vi "Read Configure.vi"(8 "error in (no error)":errorcluster, 11 "Gluing Procedure in":refnum<class "Gluing Procedure.lvclass">) -> (0 "error out":errorcluster, 2 "Configure":T1={"Has been run?"=FALSE, "Active Paths"=[TRUE, TRUE, TRUE, TRUE], "Glue Pathways"=[{"HDI Slot "=0, "Stamp Slot"=0, "Glue Slot"=0, "Weight Slot"=0, "BBM Slot"=0}, {"HDI Slot "=1, "Stamp Slot"=1, "Glue Slot"=1, "Weight Slot"=1, "BBM Slot"=1}, {"HDI Slot "=2, "Stamp Slot"=2, "Glue Slot"=2, "Weight Slot"=2, "BBM Slot"=2}, {"HDI Slot "=3, "Stamp Slot"=3, "Glue Slot"=3, "Weight Slot"=3, "BBM Slot"=3}], "Chuck Module Used for BBM:"=0} {"Chuck Module Used for BBM:" items=["Chuck 1", "Chuck 2", "Chuck 3", "Chuck 4"]; "Glue Pathways"."BBM Slot" items=["Slot 1", "Slot 2", "Slot 3", "Slot 4"]; "Glue Pathways"."Weight Slot" items=["Slot 1", "Slot 2", "Slot 3", "Slot 4"]; "Glue Pathways"."Glue Slot" items=["Slot 1", "Slot 2", "Slot 3", "Slot 4"]; "Glue Pathways"."Stamp Slot" items=["Slot 1", "Slot 2", "Slot 3", "Slot 4"]; "Glue Pathways"."HDI Slot" items=["Slot 1", "Slot 2", "Slot 3", "Slot 4"]}, 3 "Gluing Procedure out":refnum<class "Gluing Procedure.lvclass">)   [LabVIEW 2011, in "Gluing Procedure.lvclass"]
uses:
  Gluing Procedure.lvclass
  Type Definitions/Configure.ctl
  UI typedefs/Active Paths.ctl
  UI typedefs/Glue Paths.ctl
  UI typedefs/Glue Path.ctl
  UI typedefs/BBM Chuck Used.ctl
  Gluing Procedure.lvclass/Gluing Procedure.ctl
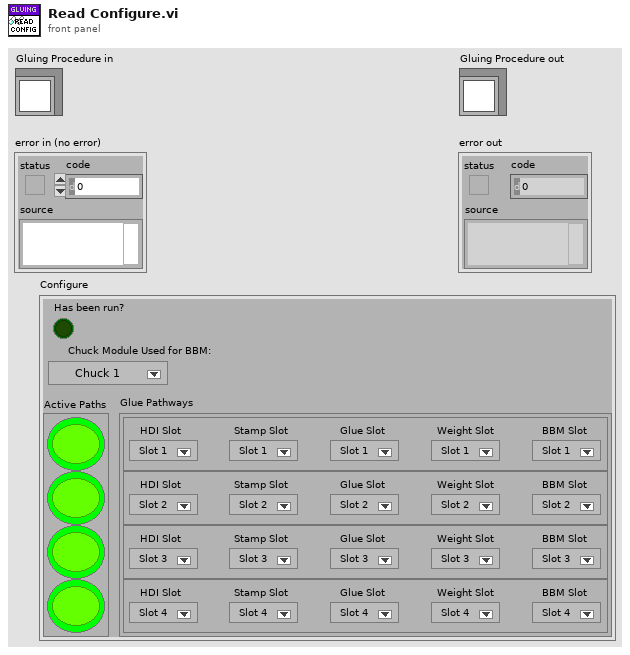
[diagram p1: front panel]
types:
  T1 = typedef "Configure.ctl" = cluster{"Has been run?":bool, "Active Paths":T2, "Glue Pathways":T3, "Chuck Module Used for BBM:":T5}
  T2 = typedef "Active Paths.ctl" = bool[]
  T3 = typedef "Glue Paths.ctl" = T4[]
  T4 = typedef "Glue Path.ctl" = cluster{"HDI Slot ":i32, "Stamp Slot":i32, "Glue Slot":i32, "Weight Slot":i32, "BBM Slot":i32}
  T5 = typedef "BBM Chuck Used.ctl" = i32
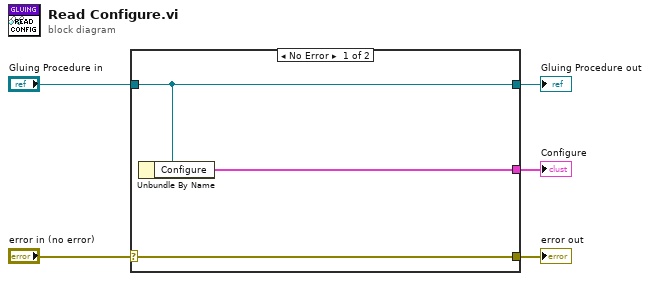
[diagram p0: block diagram]
diagram:
  n1 = case shown="No Error" "error in (no error)" {
    selector: "error in (no error)" -> [w8 w9]
    tunnel: [w8 w9] -> w4
    tunnel: [w7 w10] -> w2
    tunnel: "Gluing Procedure in" -> [w7 w10]
    tunnel: [w6 _] -> w1
    frame No Error {
      n2 = Unbundle By Name(w7) -> ("Configure"=w6:T1)
    }
    frame Error {
    }
  }
  "error out" <- w4
  "Gluing Procedure out" <- w2
  "Configure" <- w1
